vi "FahrzustandSchaltung.vi"(4 "Sensoren":dbl[](array[numeric]), 5 "Geschwindigkeitsmultiplikator":dbl, 7 "Fahrzustand":T1) -> (0 "PWM Motor":dbl, 1 "PWM Lenkung":dbl, 2 "Rundenzeiten":dbl[](array[numeric]), 3 "Linefollow_Array":bool[](array[boolean]))   [LabVIEW 2016]
uses:
  Control/Fahrart.ctl
  <vilib>/myRIO/Instrument Drivers/Onboard IO/DIO/typedefs/DIO Reference.ctl
  <vilib>/myRIO/Common/Instrument Driver Framework/Utilities/typedefs/myRIO Generic Hardware Reference.ctl
  <vilib>/myRIO/Common/Instrument Driver Framework/Utilities/typedefs/Hardware Version Enum.ctl
  <vilib>/myRIO/Common/Instrument Driver Framework/Utilities/typedefs/myRIO v1.0 Reference.ctl
  <vilib>/myRIO/Common/Instrument Driver Framework/Utilities/typedefs/Generic FPGA Reference.ctl
  <vilib>/myRIO/Common/Instrument Driver Framework/myRIO v1.0/DIO/typedefs/DIO Channels List.ctl
  <vilib>/myRIO/Common/Instrument Driver Framework/myRIO v1.0/DIO/typedefs/DIO Channels Enum.ctl
  <vilib>/userdefined/High Color/nirio_resource_hc.ctl
  <vilib>/myRIO/Common/Instrument Driver Framework/Utilities/vis/Is FPGA Ref Available.vi
  <vilib>/myRIO/Common/Instrument Driver Framework/myRIO v1.0/DIO/vis/myRIO v1.1 Open DIO.vi
  <vilib>/myRIO/Instrument Drivers/Onboard IO/DIO/vis/Write.vi
  <vilib>/myRIO/Common/Instrument Driver Framework/Utilities/vis/Validate Channels.vi
  <vilib>/myRIO/Common/Instrument Driver Framework/myRIO v1.0/DIO/vis/myRIO v1.0 Reserve DIO.vi
  <vilib>/myRIO/Common/Instrument Driver Framework/myRIO v1.0/Resource Manager/vis/myRIO v1.0 Reserve Channel List.vi
  <vilib>/myRIO/Common/Instrument Driver Framework/myRIO v1.0/DIO/vis/myRIO v1.0 Build MUX Configuration DIO.vi
  <vilib>/myRIO/Common/Instrument Driver Framework/myRIO v1.0/Resource Manager/vis/myRIO v1.0 Reserve Channel.vi
  <vilib>/myRIO/Common/Instrument Driver Framework/myRIO v1.0/Resource Manager/vis/myRIO v1.0 Unreserve Channel.vi
  <vilib>/myRIO/Common/Instrument Driver Framework/myRIO v1.0/Resource Manager/vis/myRIO v1.0 Create Configuration List.vi
  <vilib>/myRIO/Common/Instrument Driver Framework/myRIO v1.0/Resource Manager/vis/myRIO v1.0 Build Mutex Name.vi
  <vilib>/Utility/VariantDataType/GetNumericInfo.vi
  <vilib>/Utility/error.llb/Error Cluster From Error Code.vi
  <vilib>/myRIO/Common/Instrument Driver Framework/myRIO v1.0/myRIO v1.1 Open.vi
  <vilib>/myRIO/Common/Instrument Driver Framework/Utilities/vis/IO Manager.vi
  <vilib>/myRIO/Common/Instrument Driver Framework/Utilities/vis/Configuration Manager.vi
  <vilib>/myRIO/Common/Instrument Driver Framework/myRIO v1.0/Resource Manager/vis/myRIO v1.0 Configure IO.vi
  <vilib>/myRIO/Common/Instrument Driver Framework/myRIO v1.0/myRIO v1.0 Close.vi
  <vilib>/myRIO/Common/Instrument Driver Framework/myRIO v1.0/DIO/vis/myRIO v1.0 Write DIO.vi
  <vilib>/myRIO/Express VI/Onboard IO/DO/DO Express VI.xnode
  <vilib>/myRIO/Instrument Drivers/Onboard IO/DIO/vis/myRIO DIO Open.xnode
  <vilib>/myRIO/Instrument Drivers/Onboard IO/DIO/DIO.lvlib
panel:
  out "überholstrecke":bool
  in  "überholen":bool
  out "Position Strecke":dbl
  out "Back to Folgen":bool
  out "FollowTime":timestamp
  out "SetTimeStamp?":bool=TRUE
  out "Überholstrecke?":bool
  # "Muss default mässig true sein !"
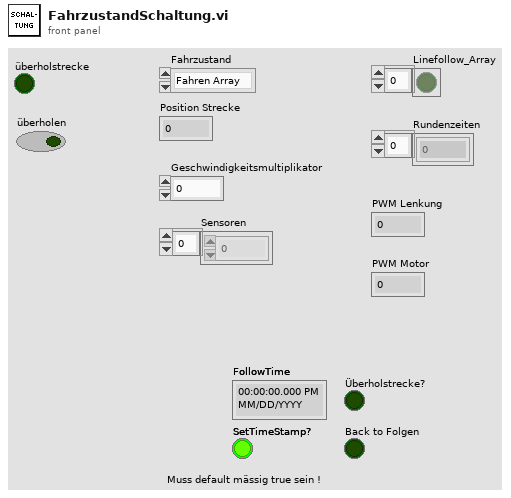
[diagram p1: front panel]
types:
  T1 = typedef "Fahrart.ctl" = enum16{"Fahren Array", "Folgen", "Überholen"}
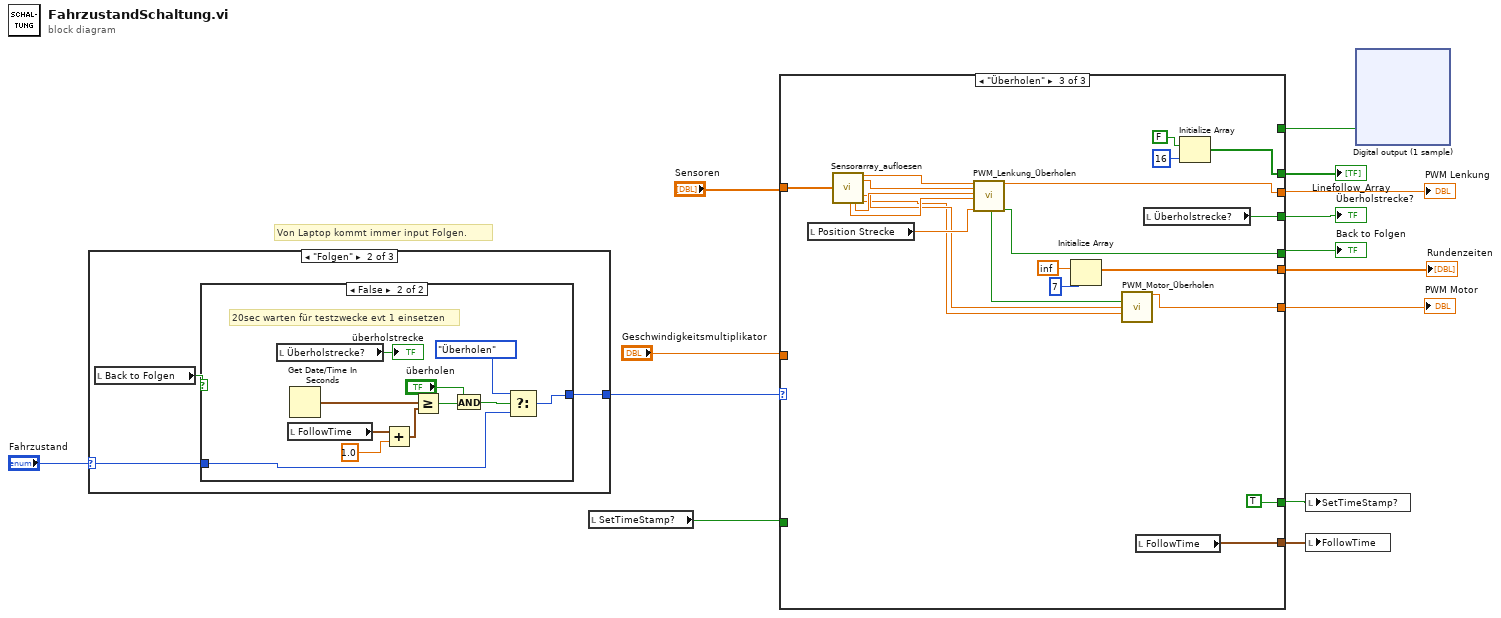
[diagram p0: block diagram]
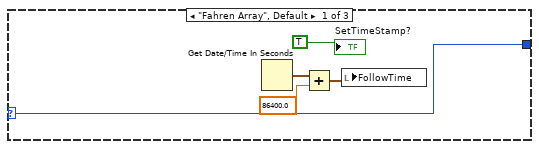
[diagram p2: hidden frame]
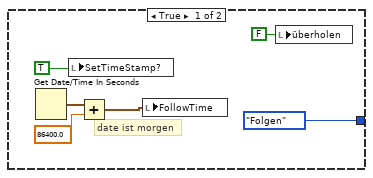
[diagram p3: hidden frame]
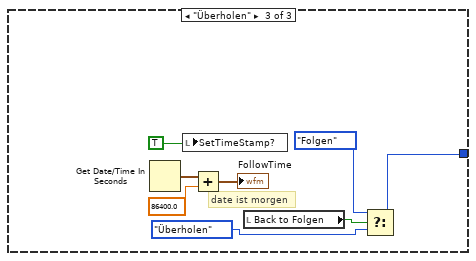
[diagram p4: hidden frame]
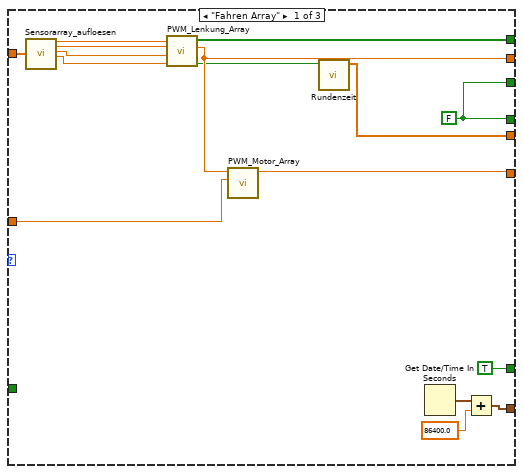
[diagram p5: hidden frame]
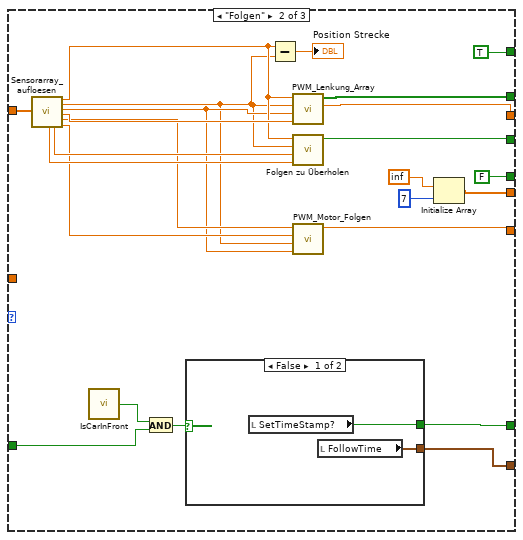
[diagram p6: hidden frame]
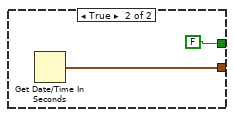
[diagram p7: hidden frame]
diagram:
  # "Von Laptop kommt immer input Folgen."
  n1 = case shown="\"Folgen\"" "Fahrzustand" {
    selector: "Fahrzustand" -> [w19 w22 _]
    tunnel: [w19 w21 w43] -> w6
    frame "Fahren Array", Default {
      n2 = Get Date/Time In Seconds() -> (seconds since 1Jan1904=w18:timestamp)
      n3 = Add(x=w18, y=86400.0) -> (x+y=w16:timestamp)
      n4 = local write "FollowTime"(w16) -> ()
      "SetTimeStamp?" <- TRUE
    }
    frame "Folgen" {
      n5 = local read "Back to Folgen"() -> (w20:bool)
      n6 = case shown="False" w20 {
        tunnel: w22 -> [_ w39]
        tunnel: [Fahrart."Folgen" ("t") w38] -> w21
        frame True {
          # "date ist morgen"
          n7 = Get Date/Time In Seconds() -> (seconds since 1Jan1904=w28:timestamp)
          n8 = local write "SetTimeStamp?"(TRUE) -> ()
          n9 = Add(x=w28, y=86400.0) -> (x+y=w25:timestamp)
          n10 = local write "FollowTime"(w25) -> ()
          n11 = local write "überholen"(FALSE ("überholen")) -> ()
        }
        frame False {
          # "20sec warten für testzwecke evt 1 einsetzen"
          n12 = local read "Überholstrecke?"() -> (→"überholstrecke":bool)
          n13 = local read "FollowTime"() -> (w33:timestamp)
          n14 = Get Date/Time In Seconds() -> (seconds since 1Jan1904=w35:timestamp)
          n15 = Add(x=w33, y=1.0) -> (x+y=w36:timestamp)
          n16 = Greater Or Equal?(x=w35, y=w36) -> (x >= y?=w29:bool)
          n17 = And(x="überholen", y=w29) -> (x .and. y?=w32:bool)
          n18 = Select(t=Fahrart."Überholen" ("Enum"), s=w32, f=w39) -> (s? t:f=w38:T1)
        }
      }
    }
    frame "Überholen" {
      # "date ist morgen"
      n19 = Get Date/Time In Seconds() -> (seconds since 1Jan1904=w47:timestamp)
      n20 = local write "SetTimeStamp?"(TRUE) -> ()
      n21 = Add(x=w47, y=86400.0) -> (x+y=→"FollowTime":timestamp)
      n22 = local read "Back to Folgen"() -> (w42:bool)
      n23 = Select(t=Fahrart."Folgen", s=w42, f=Fahrart."Überholen" ("t")) -> (s? t:f=w43:T1)
    }
  }
  n24 = local read "SetTimeStamp?"() -> (w7:bool)
  n25 = case shown="\"Überholen\"" w6 {
    tunnel: "Geschwindigkeitsmultiplikator" -> [w62 _ _]
    tunnel: [w61 w87 w112] -> w10
    tunnel: [w63 w85 w111] -> w9
    tunnel: [w53 w77 w105] -> w12
    tunnel: [w60 w86 w104] -> w11
    tunnel: w7 -> [_ w83 _]
    tunnel: "Sensoren" -> [w48 w72 w99]
    tunnel: [TRUE w82 TRUE] -> w5
    tunnel: [w56 w81 w107] -> w4
    tunnel: [w55 FALSE ("Back to Folgen") w109] -> w8
    tunnel: [w55 w80 w108] -> w3
    tunnel: [_ TRUE _] -> w2
    frame "Fahren Array" {
      w55 = FALSE
      n26 = call "Sensorarray_aufloesen.vi"("Array"=w48) -> (14:w52:dbl, "vorne links"=w51:dbl, "schräg rechts"=w50:dbl, "schräg links"=w49:dbl)  [unwired: 11 in, 4 out]
      n27 = call "PWM_Lenkung_Array.vi"("schräg links"=w49, "schräg rechts"=w50, "vorne links"=w51, "vorne rechts"=w52) -> ("16 IR true"=w54:bool, "PWM Lenkung"=w63:dbl, "Linefollow_Array"=w60:bool[])  [unwired: 4 in]
      n28 = call "PWM_Motor_Array.vi"("Geschwindigkeit\nmultiplikator"=w62, "PWM Sensor"=w63) -> ("PWM Motor"=w61:dbl)  [unwired: 9 in]
      n29 = call "Rundenzeit.vi"("8 IR true"=w54) -> ("Rundenzeiten"=w53:dbl[])  [unwired: 10 in]
      n30 = Get Date/Time In Seconds() -> (seconds since 1Jan1904=w58:timestamp)
      n31 = Add(x=w58, y=86400.0) -> (x+y=w56:timestamp)
    }
    frame "Folgen" {
      n32 = call "Sensorarray_aufloesen.vi"("Array"=w72) -> ("hinten links"=w68:dbl, "hinten rechts"=w69:dbl, 14:w70:dbl, "vorne links"=w64:dbl, "schräg rechts"=w65:dbl, "schräg links"=w71:dbl, "gerade rechts"=w67:dbl, "gerade links"=w66:dbl)  [unwired: 11 in]
      n33 = call "IsCarInFront.vi"() -> ("IsFollowingAuto"=w79:bool)  [unwired: 2 in]
      n34 = And(x=w79, y=w83) -> (x .and. y?=w84:bool)
      n35 = case shown="False" w84 {
        tunnel: [w89 FALSE] -> w82
        tunnel: [w88 w90] -> w81
        frame False {
          n36 = local read "SetTimeStamp?"() -> (w89:bool)
          n37 = local read "FollowTime"() -> (w88:timestamp)
        }
        frame True {
          n38 = Get Date/Time In Seconds() -> (seconds since 1Jan1904=w90:timestamp)
        }
      }
      n39 = Subtract(x=w70, y=w64) -> (x-y=→"Position Strecke":dbl)
      n40 = call "PWM_Lenkung_Array.vi"("schräg links"=w71, "schräg rechts"=w65, "vorne links"=w64, "vorne rechts"=w70) -> ("PWM Lenkung"=w85:dbl, "Linefollow_Array"=w86:bool[])  [unwired: 4 in, 1 out]
      n41 = call "Folgen zu Überholen.vi"("hinten links"=w68, "hinten rechts"=w69, "vorne links"=w64, "vorne rechts"=w70) -> ("Überholstrecke?"=w80:bool)  [unwired: 7 in]
      n42 = call "PWM_Motor_Folgen.vi"("Sensor gerade rechts"=w67, "Sensor gerade links"=w66, "Sensor schräg rechts"=w64, "Sensor schräg links"=w65) -> ("PWM Motor"=w87:dbl)  [unwired: 6 in]
      n43 = Initialize Array(inf, 7 ("dimension size")) -> (w77:dbl[])
    }
    frame "Überholen" {
      n44 = local read "Position Strecke"() -> (w100:dbl)
      n45 = call "Sensorarray_aufloesen.vi"("Array"=w99) -> ("hinten links"=w95:dbl, "hinten rechts"=w96:dbl, 14:w98:dbl, "vorne links"=w97:dbl, "gerade rechts"=w94:dbl, "gerade links"=w93:dbl)  [unwired: 11 in, 2 out]
      n46 = call "PWM_Lenkung_Überholen.vi"("vorne rechts"=w98, "vorne links"=w97, "hinten rechts"=w96, "hinten links"=w95, "Position Strecke"=w100) -> ("Abstand Bande erreicht"=w92:bool, "PWM Lenkung"=w111:dbl, "Back to Folgen"=w109:bool)  [unwired: 12 in]
      n47 = Initialize Array(inf, 7 ("dimension size")) -> (w105:dbl[])
      n48 = call "PWM_Motor_Überholen.vi"("Boolean"=w92, "Sensor geradeaus rechts"=w94, "Sensor geradeaus links"=w93) -> ("PWM Motor"=w112:dbl)  [unwired: 12 in]
      n49 = local read "FollowTime"() -> (w107:timestamp)
      n50 = local read "Überholstrecke?"() -> (w108:bool)
      n51 = Initialize Array(FALSE, 16 ("dimension size")) -> (w104:bool[])
    }
  }
  "Rundenzeiten" <- w12
  "Linefollow_Array" <- w11
  "PWM Motor" <- w10
  "PWM Lenkung" <- w9
  "Back to Folgen" <- w8
  "Überholstrecke?" <- w3
  n52 = local write "SetTimeStamp?"(w5) -> ()
  n53 = local write "FollowTime"(w4) -> ()
  n54 = xnode "Digital output (1 sample)"("A/DIO9 (Pin 29)"=w2) -> ()  [unwired: 1 in, 1 out]
